vi "Get Output Dir Path.vi"() -> (1 "Example/Output/ Dir":path)   [LabVIEW 2025]
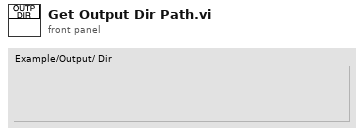
[diagram p1: front panel]
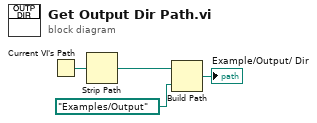
[diagram p0: block diagram]
diagram:
  n1 = Current VI's Path() -> (path=w2:path)
  n2 = Strip Path(path=w2) -> (stripped path=w1:path)  [unwired: 1 out]
  n3 = Build Path(base path=w1, name or relative path=path "Examples/Output") -> (appended path=→"Example/Output/ Dir":path)
